vi "更新调试流程.vi"   [LabVIEW 2016, in "斯坦道通用流路CODmn.lvlib"]
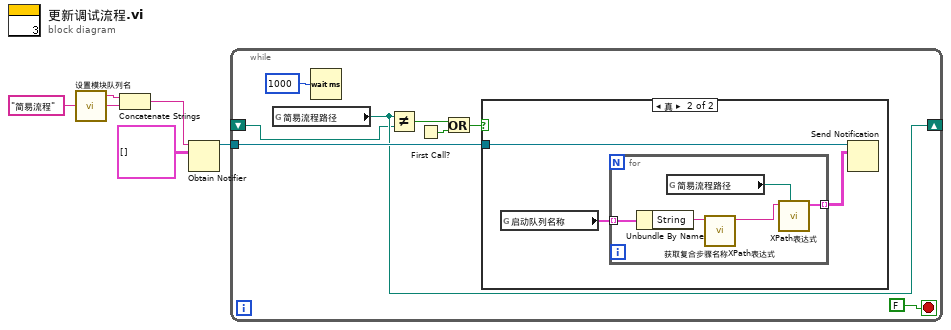
[diagram p0: block diagram]
diagram:
  n1 = call "设置模块队列名.vi"() -> ("Msg"=w3:string)  [unwired: 5 in]
  n2 = Concatenate Strings(w3, "简易流程" ("Msg")) -> (w1:string)
  n3 = Obtain Notifier(name (unnamed)=w1, notification data type=cluster{string, i32}[][] [] ("数组")) -> (notifier out=w5:refnum<notifier>)  [unwired: 2 in, 2 out]
  n4 = while {
    tunnel: w5 -> [w11]
    shift-right: [w10] -> _
    shift-left: _ -> [w9]
    stop <- FALSE stop-if-true
    n5 = global read "总磷总氮断电保存全局变量.vi" "简易流程路径"() -> (w10:path)
    n6 = Wait (ms)(milliseconds to wait=u32 1000 ("等待时间（毫秒）")) -> ()  [unwired: 1 out]
    n7 = Not Equal?(x=w10, y=w9) -> (x != y?=w8:bool)
    n8 = First Call?() -> (First Call?: T/F=w7:bool)
    n9 = Or(x=w8, y=w7) -> (x .or. y?=w6:bool)
    n10 = case shown="真" w6 {
      tunnel: w11 -> [_ w15]
      frame False {
      }
      frame True {
        n11 = global read "model config var.vi" "启动队列名称"() -> (w16:cluster{"String":string, "Value":u16}[])
        n12 = for {
          tunnel: w16 -> [w19] mode=indexing
          tunnel: [w17] -> w14 mode=indexing
          n13 = Unbundle By Name(w19) -> ("String"=w18:string)
          n14 = global read "总磷总氮断电保存全局变量.vi" "简易流程路径"() -> (w20:path)
          n15 = call "获取复合步骤名称XPath表达式.vi"("查询参数"=w18) -> ("Union"=w21:string)  [unwired: 10 in]
          n16 = call "XPath表达式.vi"("添加的路径"=w20, "XPath expression"=w21) -> ("数组"=w17:cluster{string, i32}[])  [unwired: 9 in]
        }
        n17 = Send Notification(notification=w14, notifier=w15) -> ()  [unwired: 1 in, 2 out]
      }
    }
  }
